vi "Entry Console View.vi"(8 "error in (no error)":errorcluster, 11 "View Model":T2) -> (0 "error out":errorcluster, 3 "View Model":T2)   [LabVIEW 2017]
doc: "Represent GUI for acquire CarWash steps from user"
uses:
  View Model/Controls/View Model.ctl
  Configuration Database/Controls/Config Model.ctl
  Configuration Database/Controls/Congif Data.ctl
  Configuration Database/Controls/Config Commands.ctl
  View Model/Controls/Shared Model.ctl
  Error Handler/Controls/Error Model.ctl
  Error Handler/Controls/Error Data.ctl
  Error Handler/Controls/Error Type.ctl
  Car Wash Controller/Controls/Car Wash Model.ctl
  Car Wash Controller/Controls/Car Wash States.ctl
  Car Wash Controller/Controls/Controller Overhead.ctl
  Car Wash Controller/Controls/Vehicle Location.ctl
  Car Wash Controller/Controls/CarWash CMD.ctl
  Controls/Entry Console Data.ctl
panel:
  in  "Start Wash":bool
  in  "Entry Console":T1
  # "[Covers: UI2]"
  # "[Covers: UI2A]"
  # "[Covers: UI2B]"
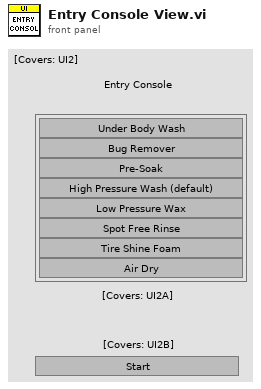
[diagram p1: front panel]
types:
  T1 = typedef "Entry Console Data.ctl" = cluster{"Under Body Wash":bool, "Bug Remover":bool, "Pre-Soak":bool, "High Pressure Wash":bool, "Low Pressure Wax":bool, "Spot Free Rinse":bool, "Tire Shine Foam":bool, "Air Dry":bool}
  T2 = typedef "View Model.ctl" = cluster{"Config Model":T3, "Shared Model":T4, "Error Model":T5, "Car Wash Model":T6}
  T3 = typedef "Config Model.ctl" = cluster{"Config Event":refnum<user-event>, "Config DVR":refnum<data-value>, "Config CMD":refnum<user-event>, "Config Locked?":refnum<data-value>}
  T4 = typedef "Shared Model.ctl" = cluster{"Stop event":refnum<user-event>, "Stop DVR":refnum<data-value>}
  T5 = typedef "Error Model.ctl" = cluster{"Error event":refnum<user-event>, "Error DVR":refnum<data-value>}
  T6 = typedef "Car Wash Model.ctl" = cluster{"State Change":refnum<user-event>, "Out of Position Change":refnum<user-event>, "Wash Entry Change":refnum<user-event>, "Contr Overhead DVR":refnum<data-value>, "Contr Overhead Event":refnum<user-event>, "CarWash CMD":refnum<user-event>, "Location Change":refnum<user-event>}
  T7 = enum8{"Enabled", "Disabled", "Disabled and Grayed Out"}
  T8 = typedef "Car Wash States.ctl" = enum16{"Initial", "Wait for start", "Start", "Wait for vehicle", "Wash Step Execution", "Wash Step Complete", "Wash Cycle Complete", "Wash Exit", "Wash Abort", "Terminate"}
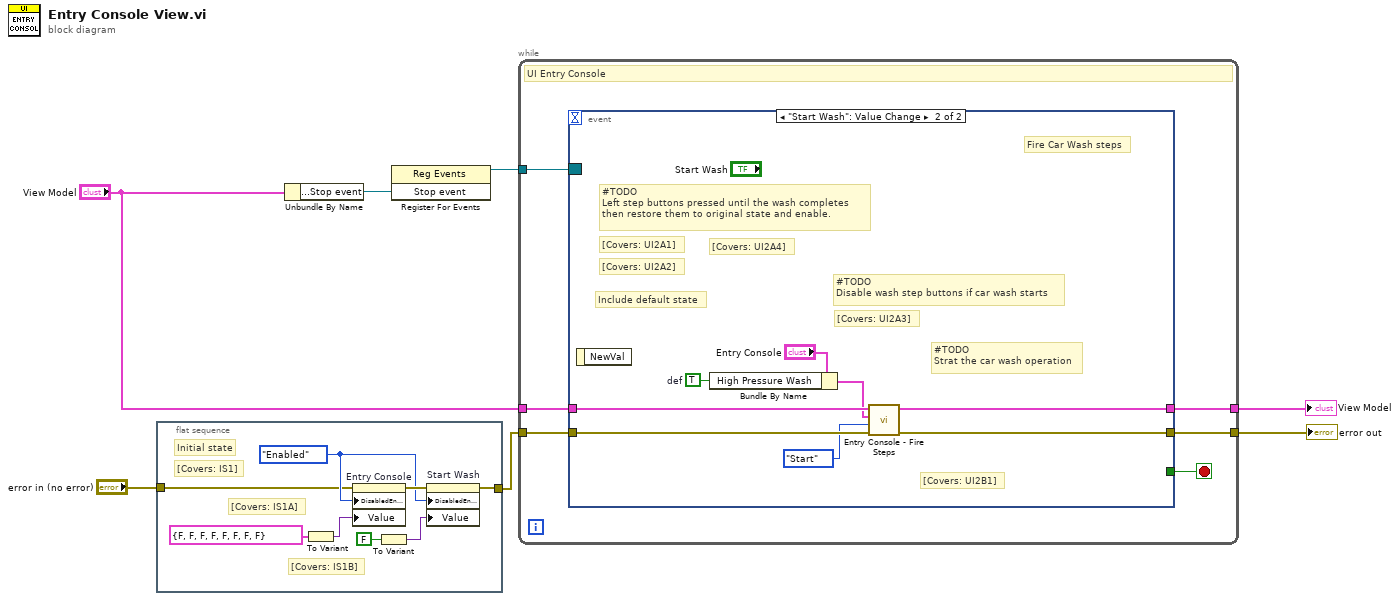
[diagram p0: block diagram]
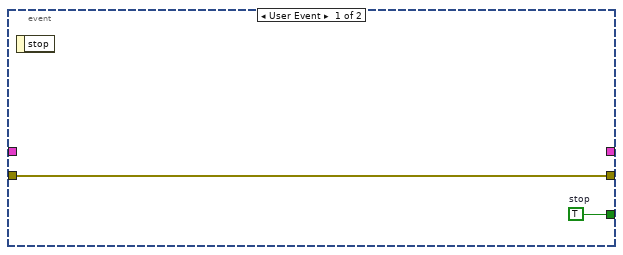
[diagram p2: hidden frame]
diagram:
  n1 = flat-sequence {
    tunnel: "error in (no error)" -> [w11]
    tunnel: [w14] -> w1
    frame #0 {
      w13 = T7."Enabled" ("Disabled")
      # "[Covers: IS1]"
      # "[Covers: IS1B]"
      # "[Covers: IS1A]"
      # "Initial state"
      n2 = To Variant(anything=T1 {"Under Body Wash"=FALSE, "Bug Remover"=FALSE, "Pre-Soak"=FALSE, "High Pressure Wash"=FALSE, "Low Pressure Wax"=FALSE, "Spot Free Rinse"=FALSE, "Tire Shine Foam"=FALSE, "Air Dry"=FALSE} ("Entry Console")) -> (Variant=w10:variant)
      n3 = property on="Entry Console" class="Clust"(error in=w11, "DisabledEnum"=w13, "Value"=w10) -> (error out=w15:errorcluster)  [unwired: 1 in, 1 out]
      n4 = To Variant(anything=FALSE ("Start Wash")) -> (Variant=w8:variant)
      n5 = property on="Start Wash" class="Bool"(error in=w15, "DisabledEnum"=w13, "Value"=w8) -> (error out=w14:errorcluster)  [unwired: 1 in, 1 out]
    }
  }
  n6 = Unbundle By Name("View Model") -> ("Shared Model.Stop event"=w5:refnum<user-event>)
  n7 = register-events(w5) -> (reference out=w7:refnum<event-registration>)  [unwired: 2 in, 1 out]
  n8 = while {
    tunnel: w7 -> [w21]
    tunnel: w1 -> [w19]
    tunnel: [w18] -> w6
    tunnel: "View Model" -> [w17]
    tunnel: [w16] -> w3
    stop <- w20 stop-if-true
    # "UI Entry Console"
    n9 = event shown="[1] \"Start Wash\": Value Change" {
      selector: w21 -> [_ _]
      dyn-events: _ -> [_ _]
      timeout: _ -> [_ _]
      tunnel: [w23 _] -> w20
      tunnel: w19 -> [w22 w31]
      tunnel: [w22 w30] -> w18
      tunnel: w17 -> [_ w29]
      tunnel: [_ w24] -> w16
      event User Event {
        w23 = TRUE  # stop
        n10 = event-data() -> ()  [unwired: 1 in, 1 out]
      }
      event "Start Wash": Value Change {
        w26 = TRUE  # def
        # "[Covers: UI2A4]"
        # "[Covers: UI2A3]"
        # "#TODO\nDisable wash step buttons if car wash starts"
        # "[Covers: UI2A2]"
        # "[Covers: UI2A1]"
        # "#TODO\nLeft step buttons pressed until the wash completes\nthen restore them to original state and enable."
        # "[Covers: UI2B1]"
        # "#TODO\nStrat the car wash operation"
        # "Include default state"
        # "Fire Car Wash steps"
        n11 = event-data() -> ()  [unwired: 1 in, 1 out]
        n12 = Bundle By Name(cluster="Entry Console", "High Pressure Wash"=w26) -> (w25:T1)
        n13 = call "Entry Console - Fire Steps.vi"("error in (no error)"=w31, "CarWash States"=Car_Wash_States."Start", "Entry Console Data"=w25, "View Model"=w29) -> ("error out"=w30:errorcluster, "View Model"=w24:T2)  [unwired: 6 in]
      }
    }
  }
  "error out" <- w6
  "View Model" <- w3
